vi "oef4.vi"() -> ()   [LabVIEW 2021]
uses:
  72b7df48-6abe-7a48-9ac6-543cd21f165a.vi
  <vilib>/Comparison/Less/Less Functor/Less Functor.lvclass
panel:
  in  "stop":bool
  out "sorted array":dbl[](array[numeric])
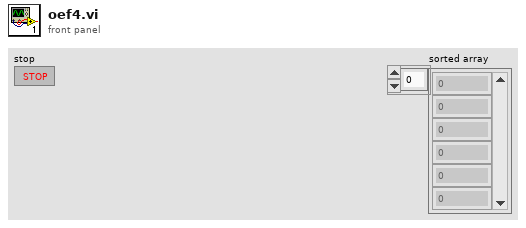
[diagram p1: front panel]
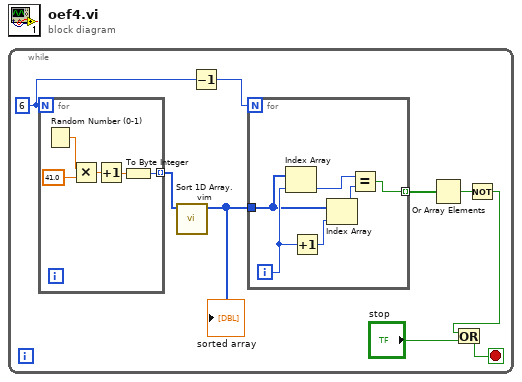
[diagram p0: block diagram]
diagram:
  n1 = while {
    stop <- w4 stop-if-true
    w6 = 6
    n2 = for {
      N: w6 -> [_]
      tunnel: [w17] -> w8 mode=indexing
      n3 = Random Number (0-1)() -> (number: 0 to 1=w20:dbl)
      n4 = Multiply(x=w20, y=41.0) -> (x*y=w18:dbl)
      n5 = Increment(x=w18) -> (x+1=w16:dbl)
      n6 = To Byte Integer(number=w16) -> (8bit integer=w17:i8)
    }
    n7 = call "Sort 1D Array.vim"("unsorted array"=w8) -> ("sorted array"=w9:i8[])  [unwired: 10 in]
    "sorted array" <- w9
    n8 = Decrement(x=w6) -> (x-1=w7:i32)
    n9 = for {
      N: w7 -> [_]
      tunnel: w9 -> [w13]
      tunnel: [w10] -> w3 mode=indexing
      i -> [w15]
      n10 = Index Array(array=w13, index=w15) -> (element=w11:i8)
      n11 = Increment(x=w15) -> (x+1=w14:i32)
      n12 = Index Array(array=w13, index=w14) -> (element=w12:i8)
      n13 = Equal?(x=w11, y=w12) -> (x = y?=w10:bool)
    }
    n14 = Or Array Elements(Boolean array=w3) -> (logical OR=w2:bool)
    n15 = Not(x=w2) -> (.not. x?=w1:bool)
    n16 = Or(x=w1, y="stop") -> (x .or. y?=w4:bool)
  }
